vi "8 channel 24-bit TDM Example Simulation.vi"() -> ()   [LabVIEW 2013]
uses:
  <vilib>/rvi/DesktopExecutionNode/Execution/niFpgaDEN_Execute.vi
  <vilib>/rvi/DesktopExecutionNode/DesktopExecutionNode.xnode
  Source/I2S-TDM.lvlib
panel:
  out "FIFO Elements":u32
  in  "Loop Wait":u32(slide)=45 min=10 max=70 step=1 scale=10.0..70.0
  in  "pause":bool
  out "Digital Waveform Graph":digitalwaveform(graph)
  in  "stop":bool
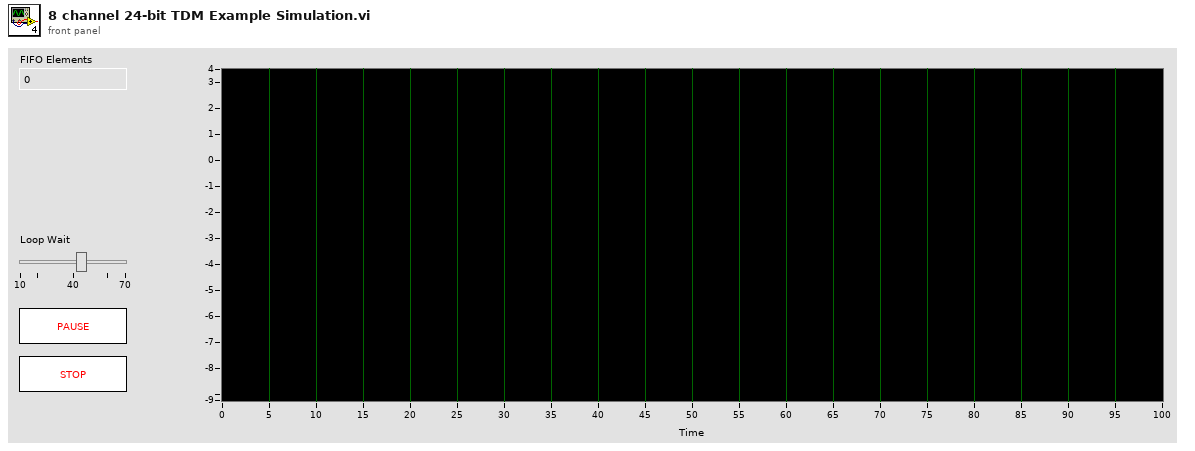
[diagram p1: front panel]
types:
  T1 = cluster{"clock":bool, "frame sync":bool, "sdata":bool}
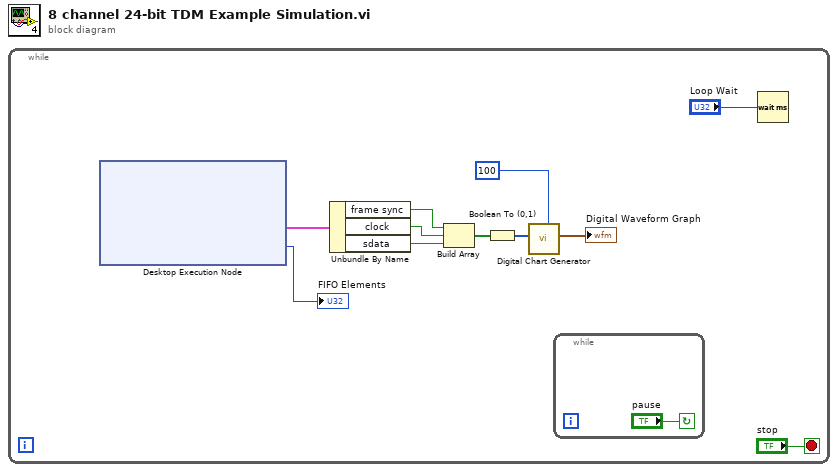
[diagram p0: block diagram]
diagram:
  n1 = while {
    stop <- "stop" stop-if-true
    n2 = xnode "Desktop Execution Node"() -> ("signals out"=w2:T1, "FIFO Elements"=→"FIFO Elements":u32)  [unwired: 1 in, 1 out]
    n3 = Unbundle By Name(w2) -> ("frame sync"=w4:bool, "clock"=w5:bool, "sdata"=w6:bool)
    n4 = Build Array(w4, w5, w6) -> (w8:bool[])
    n5 = Boolean To (0,1)(Boolean=w8) -> (0, 1=w7:i16[])
    n6 = call "Digital Chart Generator.vi"("History Size"=100, "Input"=w7) -> ("Digital Data"=→"Digital Waveform Graph":digitalwaveform)  [unwired: 9 in]
    n7 = while {
      stop <- "pause" continue-if-true
    }
    n8 = Wait (ms)(milliseconds to wait="Loop Wait") -> ()  [unwired: 1 out]
  }
